vi "AlignByKeyPress.vi"(6 "KeyChar":string, 8 "error in (no error)":errorcluster, 9 "Executed on Frontpanel?":bool, 10 "Panel Ref":refnum<vi>, 11 "TopLevelDiagram in":refnum<vi>) -> (0 "error out":errorcluster, 1 "Align Executed?":bool, 2 "Panel Ref out":refnum<vi>, 3 "TopLevelDiagram out":refnum<vi>)   [LabVIEW 2016, in "Align Elements.lvlib"]
uses:
  Align Elements.lvlib
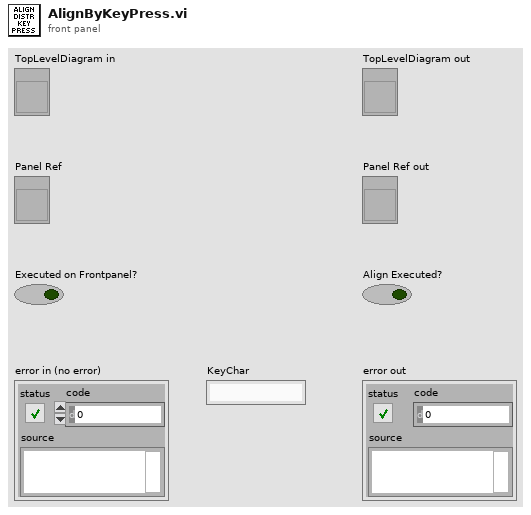
[diagram p1: front panel]
types:
  T1 = enum32{"Top Edges", "Vertical Centers", "Bottom Edges", "Left Edges", "Horizontal Centers", "Right Edges"}
  T2 = enum32{"Top Edges", "Vertical Centers", "Bottom Edges", "Vertical Gap", "Vertical Compress", "Left Edges", "Horizontal Centers", "Right Edges", "Horizontal Gap", "Horizontal Compress"}
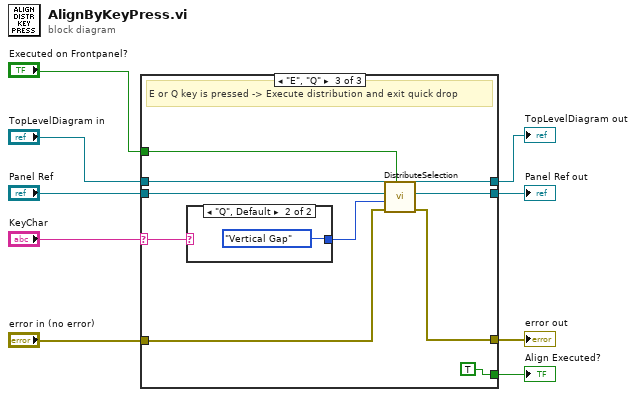
[diagram p0: block diagram]
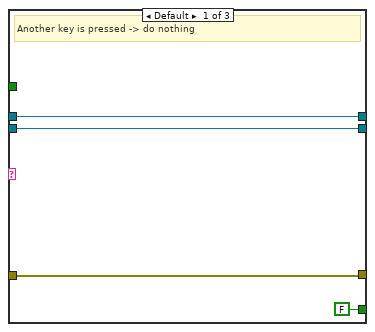
[diagram p2: hidden frame]
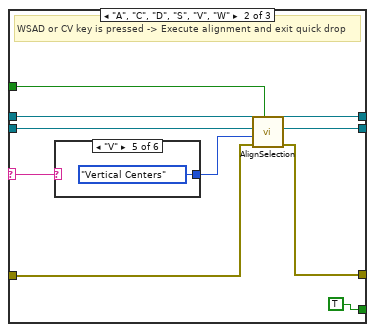
[diagram p3: hidden frame]
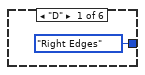
[diagram p4: hidden frame]
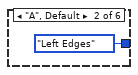
[diagram p5: hidden frame]
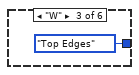
[diagram p6: hidden frame]
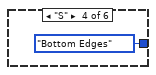
[diagram p7: hidden frame]
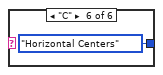
[diagram p8: hidden frame]
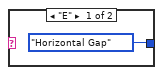
[diagram p9: hidden frame]
diagram:
  n1 = case shown="\"E\", \"Q\"" "KeyChar" {
    selector: "KeyChar" -> [_ w23 w39]
    tunnel: "TopLevelDiagram in" -> [w13 w22 w38]
    tunnel: [w13 w21 w37] -> w3
    tunnel: "Panel Ref" -> [w12 w20 w36]
    tunnel: [w12 w19 w35] -> w5
    tunnel: "error in (no error)" -> [w11 w18 w34]
    tunnel: [w11 w17 w33] -> w7
    tunnel: "Executed on Frontpanel?" -> [_ w14 w31]
    tunnel: [FALSE TRUE TRUE] -> w8
    frame Default {
      # "Another key is pressed -> do nothing"
    }
    frame "A", "C", "D", "S", "V", "W" {
      # "WSAD or CV key is pressed -> Execute alignment and exit quick drop"
      n2 = case shown="\"V\"" w23 {
        tunnel: [T1."Right Edges" ("Align Type") T1."Left Edges" ("Align Type") T1."Top Edges" ("Align Type") T1."Bottom Edges" ("Align Type") T1."Vertical Centers" ("Align Type") T1."Horizontal Centers" ("Align Type")] -> w15
        frame "D" {
        }
        frame "A", Default {
        }
        frame "W" {
        }
        frame "S" {
        }
        frame "V" {
        }
        frame "C" {
        }
      }
      n3 = call "AlignSelection.vi"("Executed on Frontpanel?"=w14, "error in (no error)"=w18, "Align Type"=w15, "Panel Ref in"=w20, "TopLevelDiagram in"=w22) -> ("error out"=w17:errorcluster, "Panel Ref out"=w19:refnum<vi>, "TopLevelDiagram out"=w21:refnum<vi>)  [unwired: 4 in]
    }
    frame "E", "Q" {
      # "E or Q key is pressed -> Execute distribution and exit quick drop"
      n4 = case shown="\"Q\", Default" w39 {
        tunnel: [T2."Horizontal Gap" ("DistributeType") T2."Vertical Gap" ("DistributeType")] -> w30
        frame "E" {
        }
        frame "Q", Default {
        }
      }
      n5 = call "DistributeSelection.vi"("Executed on Frontpanel?"=w31, "error in (no error)"=w34, "DistributeType"=w30, "Panel Ref in"=w36, "TopLevelDiagram in"=w38) -> ("error out"=w33:errorcluster, "Panel Ref out"=w35:refnum<vi>, "TopLevelDiagram out"=w37:refnum<vi>)  [unwired: 4 in]
    }
  }
  "Align Executed?" <- w8
  "error out" <- w7
  "Panel Ref out" <- w5
  "TopLevelDiagram out" <- w3
